vi "update_channel_names.vi"(0 "Active Index Start":i32, 1 "Crate":i32[](array[numeric]), 2 "Card":i32[](array[numeric]), 3 "Channel":i32[](array[numeric]), 4 "Name":string[](array[string]), 5 "error in":errorcluster, 8 "Channel Names List":path) -> (19 "error out":errorcluster)   [LabVIEW 2018]
uses:
  CAEN globals.vi
  <vilib>/Utility/file.llb/Write Delimited Spreadsheet (string).vi
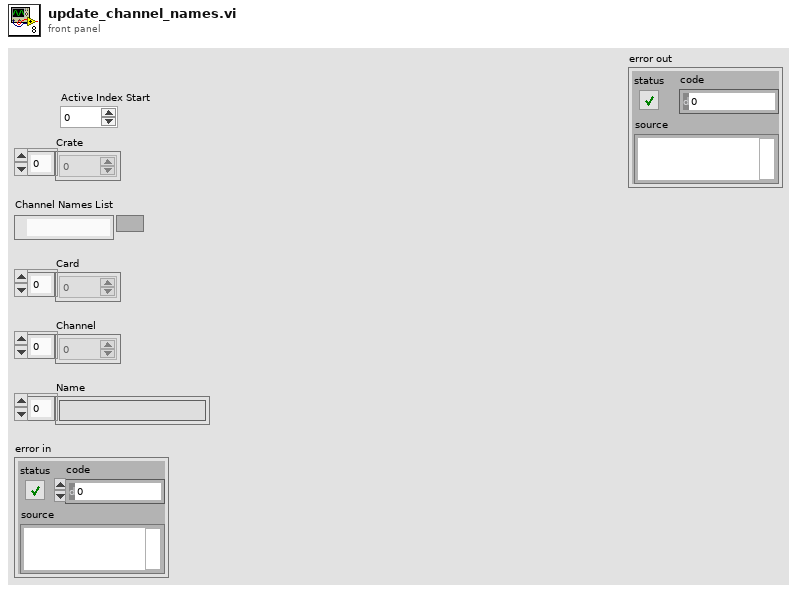
[diagram p1: front panel]
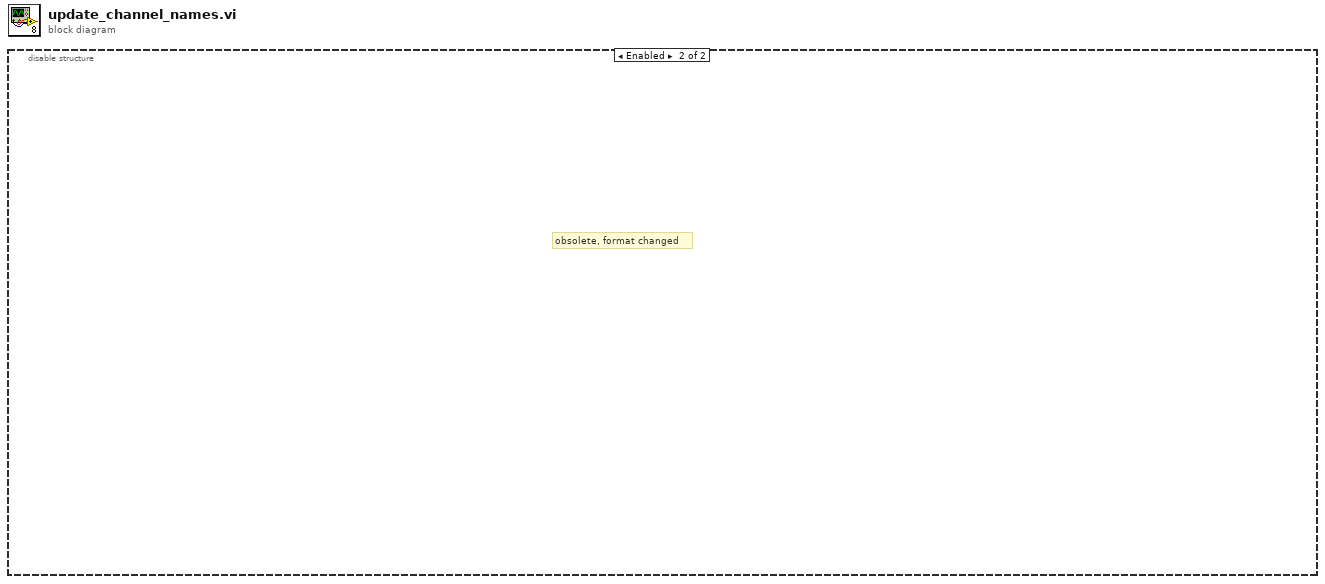
[diagram p0: block diagram]
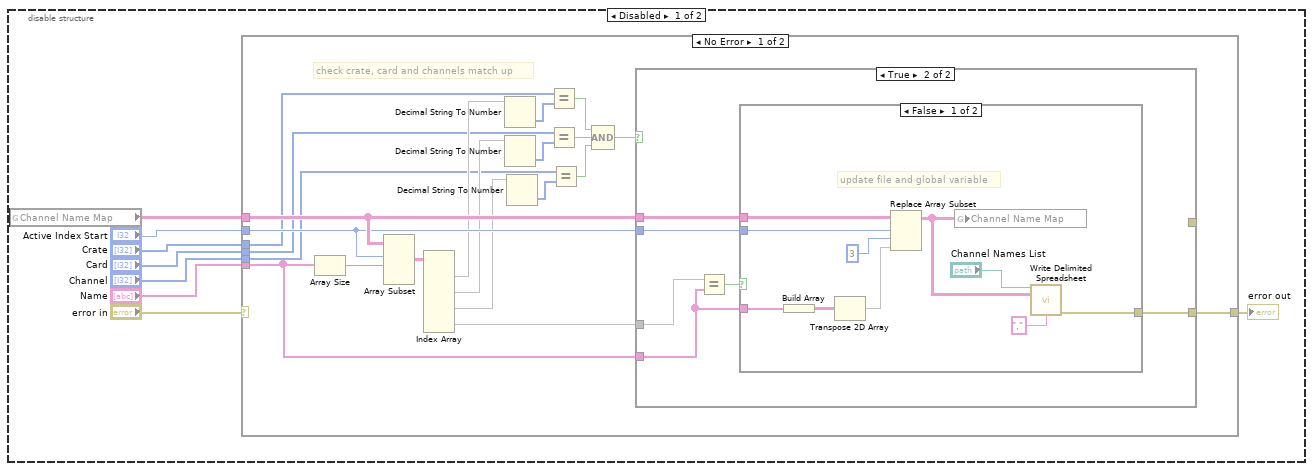
[diagram p2: hidden frame]
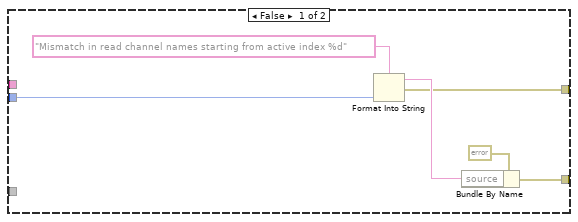
[diagram p3: hidden frame]
diagram:
  n1 = disable-structure shown="Enabled" {
    frame Disabled {
      n2 = global read "CAEN globals.vi" "Channel Name Map"() -> (w4:string[][])
      n3 = case shown="No Error" "error in" {
        selector: "error in" -> [_ w51]
        tunnel: "Active Index Start" -> [w25 _]
        tunnel: "Name" -> [w24 _]
        tunnel: "Channel" -> [w16 _]
        tunnel: "Card" -> [w20 _]
        tunnel: "Crate" -> [w21 _]
        tunnel: w4 -> [w27 _]
        tunnel: [w10 w51] -> w1
        frame No Error {
          # "check crate, card and channels match up"
          n4 = Array Size(array=w24) -> (size(s)=w9:i32)
          n5 = Array Subset(array=w27, index (row)=w25, length (row)=w9) -> (w28:string[][])  [unwired: 2 in]
          n6 = Index Array(array=w28) -> (element #1=w23:string[], element #2=w19:string[], element #3=w17:string[], element #4=w26:string[])  [unwired: 8 in]
          n7 = Decimal String To Number(string=w23) -> (number=w22:i32[])  [unwired: 2 in, 1 out]
          n8 = Decimal String To Number(string=w19) -> (number=w15:i32[])  [unwired: 2 in, 1 out]
          n9 = Decimal String To Number(string=w17) -> (number=w18:i32[])  [unwired: 2 in, 1 out]
          n10 = Equal?(x=w21, y=w22) -> (x = y?=w13:bool)
          n11 = Equal?(x=w20, y=w15) -> (x = y?=w14:bool)
          n12 = Equal?(x=w16, y=w18) -> (x = y?=w12:bool)
          n13 = Compound Arithmetic op=AND(w13, w14, w12) -> (w11:bool)
          n14 = case shown="True" w11 {
            tunnel: w27 -> [_ w39]
            tunnel: w26 -> [_ w38]
            tunnel: w25 -> [w31 w37]
            tunnel: w24 -> [_ w36]
            tunnel: [w34 w35] -> w10
            tunnel: [w29 _] -> _
            frame False {
              n15 = Format Into String(format string="Mismatch in read channel names starting from active index %d" ("source"), w31) -> (resulting string=w30:string, error out=w29:errorcluster)  [unwired: 2 in]
              n16 = Bundle By Name(cluster=errorcluster {"status"=TRUE, "code"=0, "source"=""} ("error out"), "source"=w30) -> (w34:errorcluster)
            }
            frame True {
              n17 = Equal?(x=w38, y=w36) -> (x = y?=w40:bool)
              n18 = case shown="False" w40 {
                tunnel: w39 -> [w50 _]
                tunnel: w37 -> [w48 _]
                tunnel: w36 -> [w47 _]
                tunnel: [w41 _] -> w35
                frame False {
                  # "update file and global variable"
                  n19 = Build Array(w47) -> (w46:string[][])
                  n20 = Transpose 2D Array(2D array=w46) -> (transposed array=w45:string[][])
                  n21 = Replace Array Subset(array=w50, new element=w45, index (row)=w48, index (col)=3 ("disabled index (col)")) -> (w43:string[][])
                  n22 = global write "CAEN globals.vi" "Channel Name Map"(w43) -> ()
                  n23 = call-poly <vilib>:"Write Delimited Spreadsheet.vi"("file path (dialog if empty)"="Channel Names List", "2D data"=w43, "delimiter (\\t)"="," ("delimiter (\\t)")) -> ("error out"=w41:errorcluster)  [unwired: 11 in, 1 out]
                }
                frame True {
                  # "No changes - no action"
                }
              }
            }
          }
        }
        frame Error {
        }
      }
      "error out" <- w1
    }
    frame Enabled {
      # "obsolete, format changed"
    }
  }
